vi "Graph Temperature and Setpoint.vi"() -> ()   [LabVIEW 2011]
panel:
  in  "Blinking":bool=TRUE
  out "Waveform Chart 2":cluster{dbl, dbl}(graph)
  in  "?":bool
  out "error out 2":errorcluster
  in  "error out":errorcluster
  in  "String":string
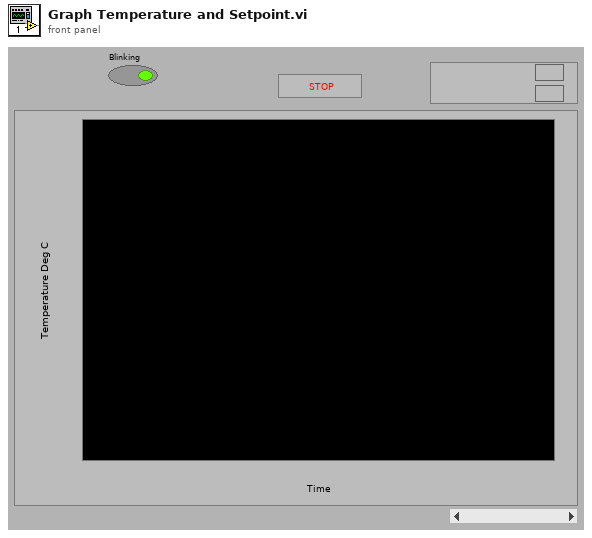
[diagram p1: front panel]
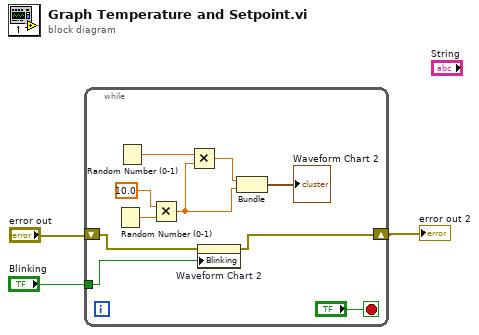
[diagram p0: block diagram]
diagram:
  n1 = while {
    shift-right: [w4] -> w3
    shift-left: "error out" -> [w5]
    tunnel: "Blinking" -> [w6]
    stop <- "?" stop-if-true
    n2 = Random Number (0-1)() -> (number: 0 to 1=w11:dbl)
    n3 = Random Number (0-1)() -> (number: 0 to 1=w12:dbl)
    n4 = Multiply(x=10.0 ("y"), y=w11) -> (x*y=w8:dbl)
    n5 = Multiply(x=w12, y=w8) -> (x*y=w10:dbl)
    n6 = property on="Waveform Chart 2" class="WFChart (strict)"(error in=w5, "Blinking"=w6) -> (error out=w4:errorcluster)  [unwired: 1 in, 1 out]
    n7 = Bundle(w10, w8) -> (→"Waveform Chart 2":cluster{dbl, dbl})  [unwired: 1 out]
  }
  "error out 2" <- w3
